vi "Teste2.vi"(10 "FPS":dbl format="%#_13g") -> ()   [LabVIEW 2022 SP3, in "Phoenix.lvclass"]
uses:
  Phoenix.lvclass
panel:
  out "COUNT":dbl format="%#_13g"
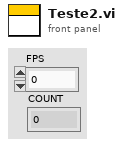
[diagram p1: front panel]
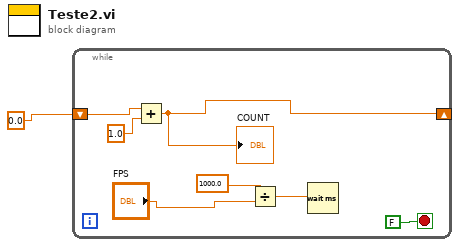
[diagram p0: block diagram]
diagram:
  n1 = while {
    shift-right: [w2] -> _
    shift-left: 0.0 -> [w4]
    stop <- FALSE stop-if-true
    n2 = Add(x=w4, y=1.0) -> (x+y=w2:dbl)
    "COUNT" <- w2
    n3 = Divide(x=1000.0, y="FPS") -> (x/y=w7:dbl)
    n4 = Wait (ms)(milliseconds to wait=w7) -> ()  [unwired: 1 out]
  }
